vi "robotTurningAroundBall.vi"(7 "Game":refnum<class "Game.lvclass">, 8 "error in (no error)":errorcluster, 9 "Target":dbl[](array[numeric]), 10 "Robot in":refnum<class "Robot.lvclass">, 11 "KickToSkill in":refnum<class "KickToSkill.lvclass">) -> (0 "error out":errorcluster, 2 "Robot out":refnum<class "Robot.lvclass">, 3 "KickToSkill out":refnum<class "KickToSkill.lvclass">)   [LabVIEW 2021, in "KickToSkill.lvclass"]
uses:
  KickToSkill.lvclass
  Game_class/Game.lvclass
  Robot_class/Robot.lvclass
  robotTurningBallStates.ctl
  Object_class/Object.lvclass/Object.ctl
  Game_class/Game.lvclass/Game.ctl
  Robot_class/Robot.lvclass/Robot.ctl
  <vilib>/Analysis/baseanly.llb/Unit Vector (DBL).vi
  <vilib>/Analysis/coordinate.llb/2D Cartesian Coordinate Rotation (Scalar).vi
  Robot_class/Read orientation.vi
  Robot_class/Read dest_orientation.vi
  Robot_class/Read dest_x.vi
  Robot_class/Read dest_y.vi
  Game_class/Read BallRef.vi
  Object_class/Read position(x,y).vi
  Object_class/Read x.vi
  Robot_class/Write dest_orientation.vi
  Robot_class/Write dest_x.vi
  Robot_class/Write dest_y.vi
  Robot_class/Write kick_x.vi
  Robot_class/Write dribble.vi
  Ball_class/Ball.lvclass
  <vilib>/Analysis/NI_AALPro.lvlib
  <vilib>/Analysis/NI_AALBase.lvlib
panel:
  in  "Raio":dbl=123.0
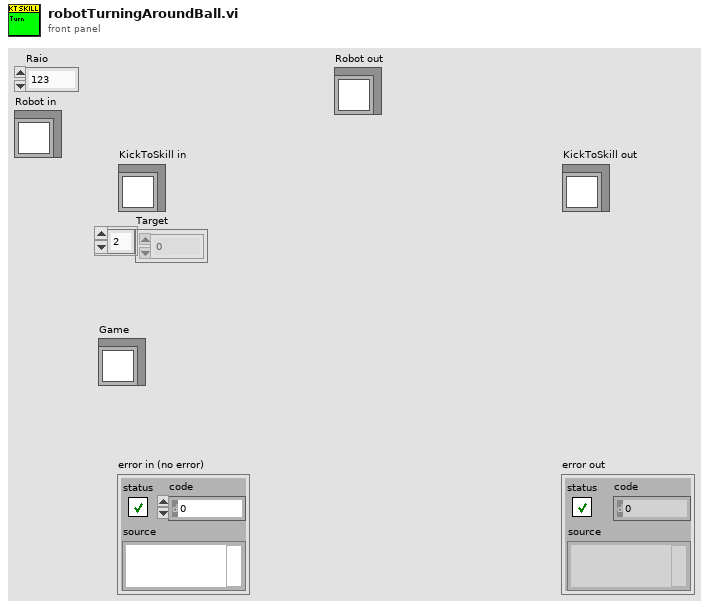
[diagram p1: front panel]
types:
  T1 = typedef "KickToSkill.lvclass/robotTurningBallStates.ctl" = enum16{"go straight to the target", "go to point A", "circulating the ball", "lining up", "shoot"}
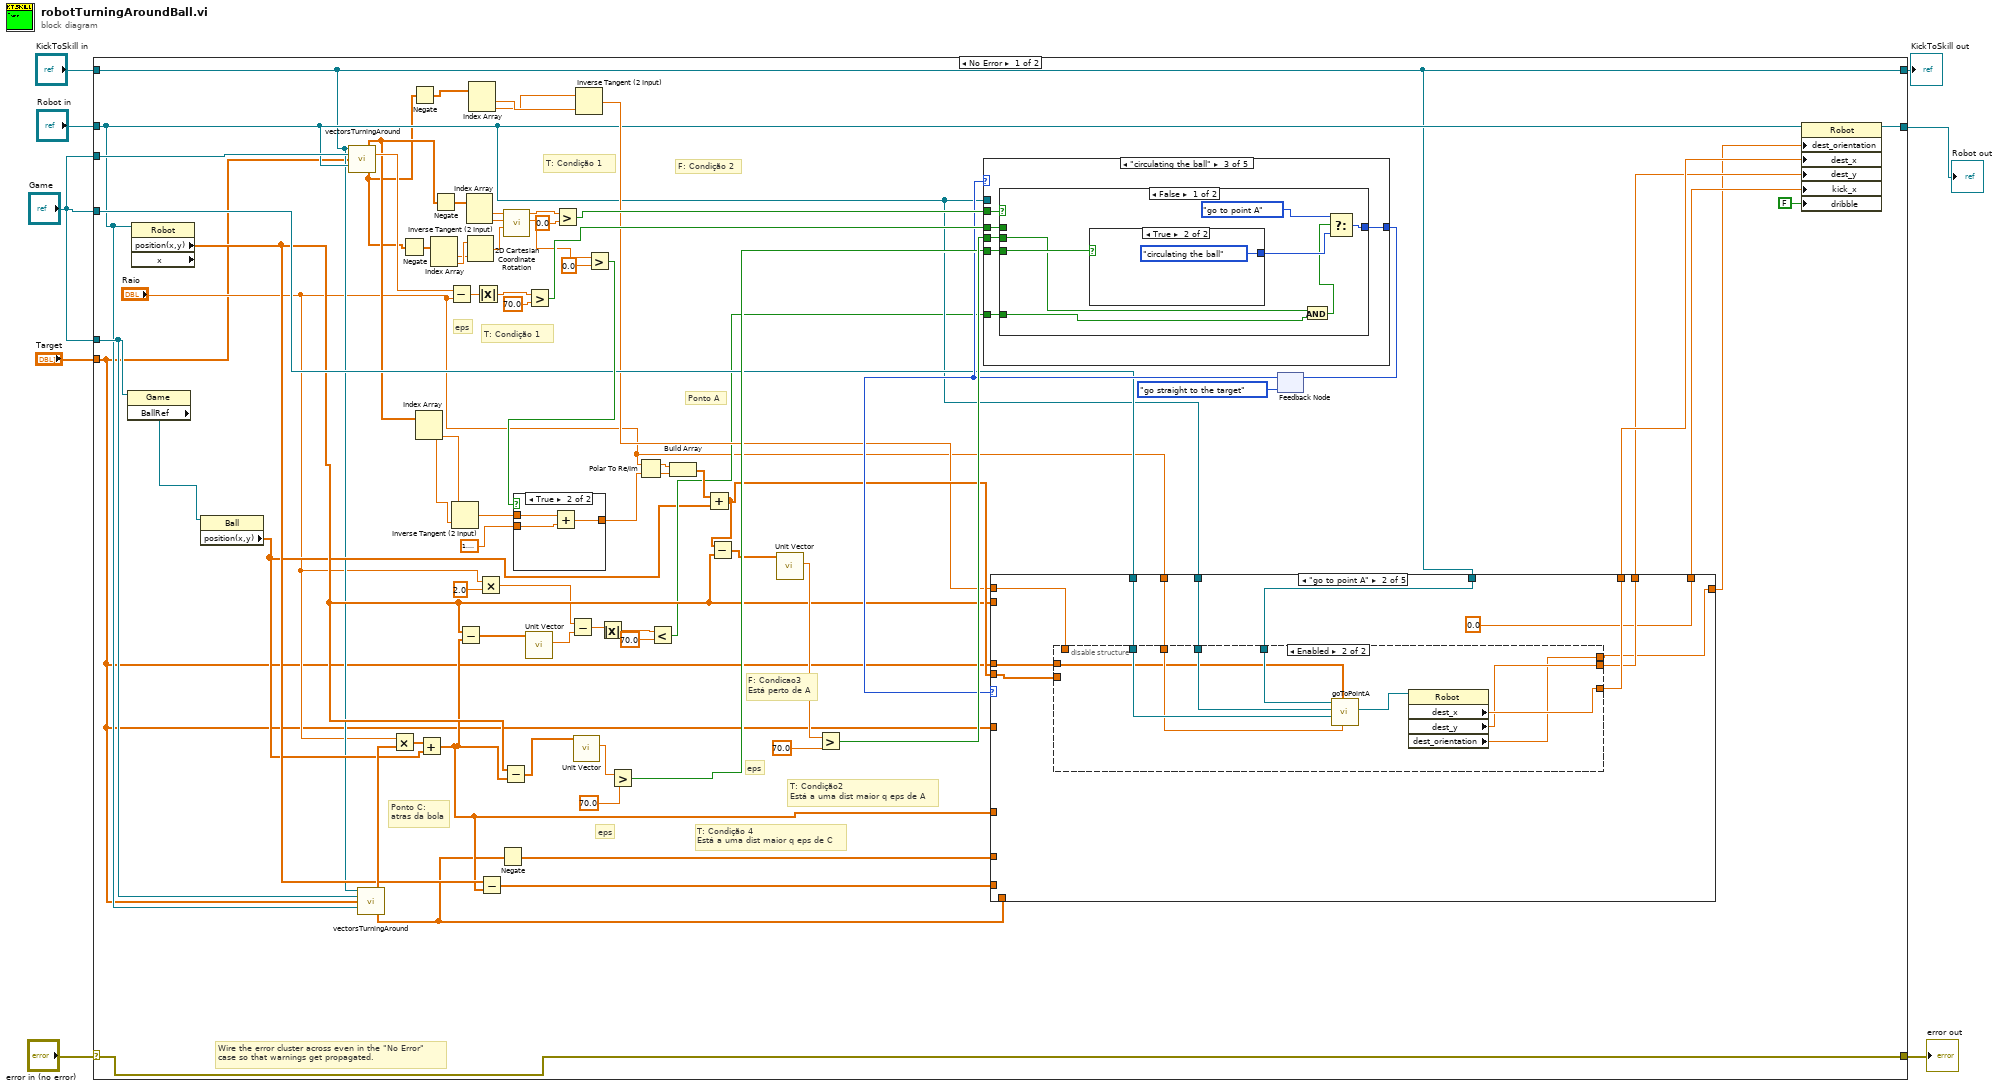
[diagram p0: block diagram]
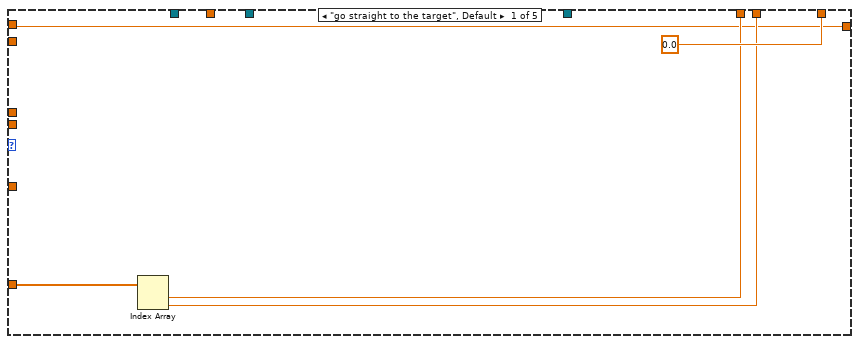
[diagram p2: hidden frame]
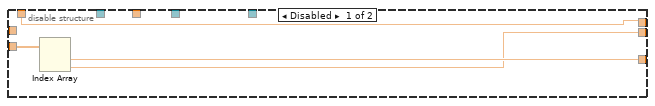
[diagram p3: hidden frame]
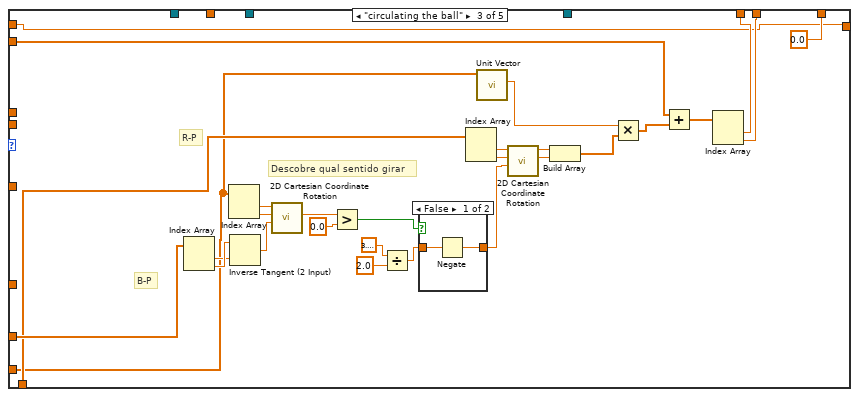
[diagram p4: hidden frame]
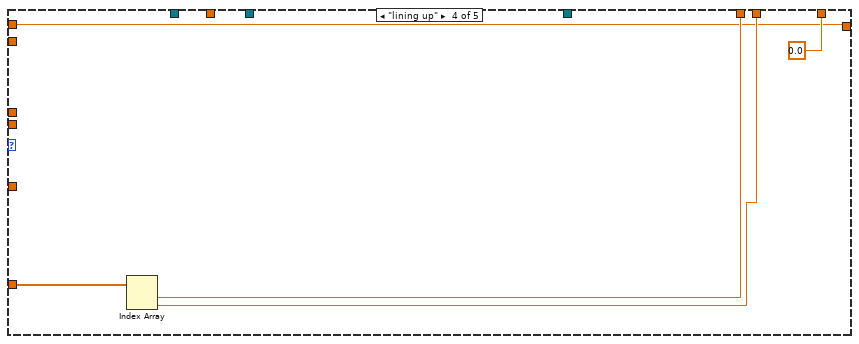
[diagram p6: hidden frame]
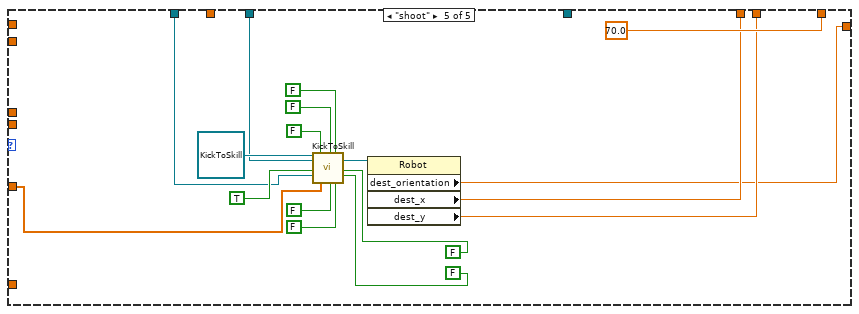
[diagram p7: hidden frame]
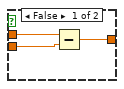
[diagram p8: hidden frame]
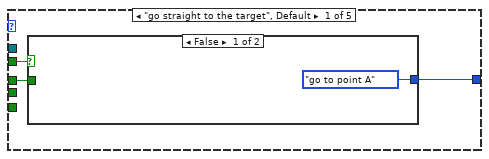
[diagram p9: hidden frame]
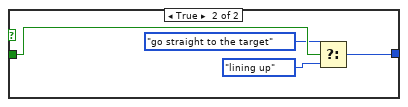
[diagram p10: hidden frame]
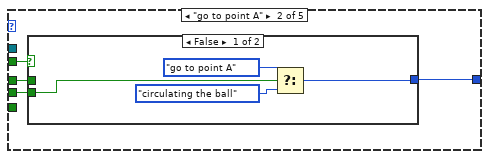
[diagram p11: hidden frame]
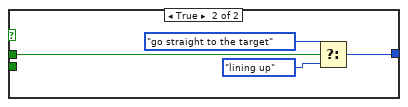
[diagram p12: hidden frame]
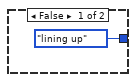
[diagram p13: hidden frame]
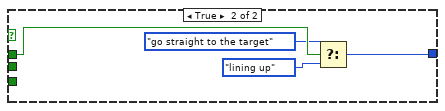
[diagram p14: hidden frame]
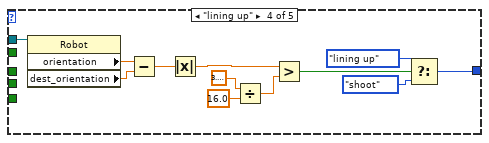
[diagram p15: hidden frame]
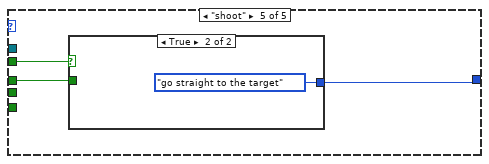
[diagram p16: hidden frame]
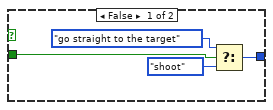
[diagram p17: hidden frame]
diagram:
  n1 = case shown="No Error" "error in (no error)" {
    selector: "error in (no error)" -> [w83 w233]
    tunnel: [w83 w233] -> w7
    tunnel: [w11 w232] -> w5
    tunnel: "KickToSkill in" -> [w11 w232]
    tunnel: "Robot in" -> [w29 w231]
    tunnel: [w82 w231] -> w3
    tunnel: "Target" -> [w9 _]
    tunnel: "Game" -> [w79 _]
    tunnel: "Game" -> [w30 _]
    tunnel: "Game" -> [w34 _]
    frame No Error {
      # "T: Condição 4\nEstá a uma dist maior q eps de C"
      # "F: Condicao3\nEstá perto de A"
      # "eps"
      # "Ponto C:\natras da bola"
      # "eps"
      # "eps"
      # "F: Condição 2"
      # "T: Condição2\nEstá a uma dist maior q eps de A"
      # "Ponto A"
      # "T: Condição 1"
      # "T: Condição 1"
      # "Wire the error cluster across even in the \"No Error\"\ncase so that warnings get propagated."
      n2 = property class="Game"(reference=w30) -> ("BallRef"=w53:refnum<class "Ball.lvclass">)  [unwired: 1 in, 2 out]
      n3 = property class="Robot" props=["position(x,y)", "x"](reference=w29) -> ("position(x,y)"=w27:dbl[])  [unwired: 1 in, 3 out]
      n4 = property class="Ball"(reference=w53) -> ("position(x,y)"=w14:dbl[])  [unwired: 1 in, 2 out]
      n5 = call "vectorsTurningAround.vi"("KickToSkill in"=w11, "Game"=w79, "Target"=w9, "Robot in"=w29) -> ("B-T"=w17:dbl[], "R-B norm"=w68:dbl, "R-B"=w16:dbl[])  [unwired: 4 in, 5 out]
      n6 = call "vectorsTurningAround.vi"("KickToSkill in"=w11, "Game"=w30, "Target"=w9, "Robot in"=w29) -> ("B-T"=w54:dbl[], "R-B"=w13:dbl[])  [unwired: 4 in, 6 out]
      n7 = Multiply(x="Raio", y=w54) -> (x*y=w52:dbl[])
      n8 = Negate(x=w16) -> (-x=w15:dbl[])
      n9 = Negate(x=w16) -> (-x=w28:dbl[])
      n10 = Index Array(array=w17) -> (element #1=w65:dbl, element #2=w64:dbl)  [unwired: 2 in]
      n11 = Add(x=w52, y=w14) -> (x+y=w26:dbl[])
      n12 = Index Array(array=w15) -> (element #1=w70:dbl, element #2=w71:dbl)  [unwired: 2 in]
      n13 = Negate(x=w17) -> (-x=w63:dbl[])
      n14 = Subtract(x=w68, y="Raio") -> (x-y=w76:dbl)
      n15 = Inverse Tangent (2 Input)(1:w65, 2:w64) -> (0:w62:dbl)
      n16 = Subtract(x=w27, y=w26) -> (x-y=w25:dbl[])
      n17 = Index Array(array=w63) -> (element #1=w72:dbl, element #2=w73:dbl)  [unwired: 2 in]
      n18 = Inverse Tangent (2 Input)(1:w70, 2:w71) -> (0:w69:dbl)
      n19 = Index Array(array=w28) -> (element #1=w41:dbl, element #2=w40:dbl)  [unwired: 2 in]
      n20 = Absolute Value(x=w76) -> (abs(x)=w77:dbl)
      n21 = Multiply(x="Raio", y=2.0) -> (x*y=w22:dbl)
      n22 = Subtract(x=w27, y=w26) -> (x-y=w35:dbl[])
      n23 = Negate(x=w13) -> (-x=w12:dbl[])
      n24 = Subtract(x=w27, y=w26) -> (x-y=w42:dbl[])
      n25 = call-poly <vilib>:"2D Cartesian Coordinate Rotation.vi"("theta"=w69, "y"=w73, "x"=w72) -> ("y out"=w60:dbl, "x out"=w74:dbl)  [unwired: 6 in, 1 out]
      n26 = call-poly <vilib>:"Unit Vector.vi"("Input Vector"=w25) -> ("norm"=w24:dbl)  [unwired: 8 in, 2 out]
      n27 = Greater?(x=w77, y=70.0) -> (0:w66:bool)
      n28 = Greater?(x=w74, y=0.0) -> (0:w67:bool)
      n29 = Subtract(x=w22, y=w24) -> (x-y=w21:dbl)
      n30 = call-poly <vilib>:"Unit Vector.vi"("Input Vector"=w42) -> ("norm"=w49:dbl)  [unwired: 8 in, 2 out]
      n31 = Inverse Tangent (2 Input)(1:w41, 2:w40) -> (0:w32:dbl)
      n32 = Greater?(x=w60, y=0.0) -> (0:w58:bool)
      n33 = case shown="True" w58 {
        tunnel: w62 -> [w167 w171]
        tunnel: 1.5707963267948966 -> [w168 w170]
        tunnel: [w166 w169] -> w47
        frame False {
          n34 = Subtract(x=w167, y=w168) -> (x-y=w166:dbl)
        }
        frame True {
          n35 = Add(x=w171, y=w170) -> (x+y=w169:dbl)
        }
      }
      n36 = Absolute Value(x=w21) -> (abs(x)=w20:dbl)
      n37 = Greater?(x=w49, y=70.0) -> (0:w50:bool)
      n38 = Polar To Re/Im(2:w47, 3:"Raio") -> (0:w45:dbl, 1:w46:dbl)
      n39 = Less?(x=w20, y=70.0) -> (x < y?=w18:bool)
      n40 = Build Array(w46, w45) -> (w44:dbl[])
      n41 = Add(x=w44, y=w14) -> (x+y=w43:dbl[])
      n42 = Subtract(x=w43, y=w27) -> (x-y=w31:dbl[])
      n43 = call-poly <vilib>:"Unit Vector.vi"("Input Vector"=w31) -> ("norm"=w56:dbl)  [unwired: 8 in, 2 out]
      n44 = Greater?(x=w56, y=70.0) -> (0:w55:bool)
      n45 = feedback #1(robotTurningBallStates."go straight to the target") -> (w48:T1)
      n46 = case shown="\"circulating the ball\"" w48 {
        tunnel: [w172 w181 w195 w211 w225] -> w81
        tunnel: w67 -> [w174 w183 w197 _ w224]
        tunnel: w66 -> [w173 w182 w196 _ w223]
        tunnel: w55 -> [_ w180 w194 _ _]
        tunnel: w50 -> [_ _ w193 _ _]
        tunnel: w29 -> [_ _ _ w222 _]
        tunnel: w18 -> [_ _ w192 _ _]
        frame "go straight to the target", Default {
          n47 = case shown="False" w174 {
            tunnel: w173 -> [_ w179]
            tunnel: [robotTurningBallStates."go to point A" w177] -> w172
            frame False {
            }
            frame True {
              n48 = Select(t=robotTurningBallStates."go straight to the target", s=w179, f=robotTurningBallStates."lining up") -> (s? t:f=w177:T1)
            }
          }
        }
        frame "go to point A" {
          n49 = case shown="False" w183 {
            tunnel: w182 -> [_ w191]
            tunnel: [w184 w189] -> w181
            tunnel: w180 -> [w187 _]
            frame False {
              n50 = Select(t=robotTurningBallStates."go to point A", s=w187, f=robotTurningBallStates."circulating the ball") -> (s? t:f=w184:T1)
            }
            frame True {
              n51 = Select(t=robotTurningBallStates."go straight to the target", s=w191, f=robotTurningBallStates."lining up") -> (s? t:f=w189:T1)
            }
          }
        }
        frame "circulating the ball" {
          n52 = case shown="False" w197 {
            tunnel: w196 -> [_ w210]
            tunnel: [w202 w208] -> w195
            tunnel: w194 -> [w200 _]
            tunnel: w193 -> [w201 _]
            tunnel: w192 -> [w199 _]
            frame False {
              n53 = case shown="True" w201 {
                tunnel: [robotTurningBallStates."lining up" robotTurningBallStates."circulating the ball"] -> w203
                frame False {
                }
                frame True {
                }
              }
              n54 = And(x=w200, y=w199) -> (x .and. y?=w198:bool)
              n55 = Select(t=robotTurningBallStates."go to point A", s=w198, f=w203) -> (s? t:f=w202:T1)
            }
            frame True {
              n56 = Select(t=robotTurningBallStates."go straight to the target", s=w210, f=robotTurningBallStates."lining up") -> (s? t:f=w208:T1)
            }
          }
        }
        frame "lining up" {
          n57 = property class="Robot"(reference=w222) -> ("orientation"=w221:dbl, "dest_orientation"=w220:dbl)  [unwired: 1 in, 2 out]
          n58 = Subtract(x=w221, y=w220) -> (x-y=w219:dbl)
          n59 = Absolute Value(x=w219) -> (abs(x)=w218:dbl)
          n60 = Divide(x=3.141592653589793, y=16.0) -> (x/y=w215:dbl)
          n61 = Greater?(x=w218, y=w215) -> (0:w214:bool)
          n62 = Select(t=robotTurningBallStates."lining up", s=w214, f=robotTurningBallStates."shoot") -> (s? t:f=w211:T1)
        }
        frame "shoot" {
          n63 = case shown="True" w224 {
            tunnel: w223 -> [w229 _]
            tunnel: [w227 robotTurningBallStates."go straight to the target"] -> w225
            frame False {
              n64 = Select(t=robotTurningBallStates."go straight to the target", s=w229, f=robotTurningBallStates."shoot") -> (s? t:f=w227:T1)
            }
            frame True {
            }
          }
        }
      }
      n65 = case shown="\"go to point A\"" w48 {
        tunnel: w43 -> [_ w99 _ _ _]
        tunnel: [0.0 ("kick_x") 0.0 ("kick_x") 0.0 ("kick_x") 0.0 ("kick_x") 70.0 ("kick_x")] -> w38
        tunnel: w26 -> [w87 _ _ w147 _]
        tunnel: [w86 w98 w115 w146 w151] -> w37
        tunnel: [w85 w97 w114 w145 w150] -> w36
        tunnel: w12 -> [_ _ w123 _ _]
        tunnel: w35 -> [_ _ w121 _ _]
        tunnel: w13 -> [_ _ w122 _ _]
        tunnel: w27 -> [_ _ w118 _ _]
        tunnel: w9 -> [_ _ _ _ w155]
        tunnel: w29 -> [_ w95 _ _ w154]
        tunnel: w34 -> [_ w94 _ _ w153]
        tunnel: w32 -> [w84 w89 w113 w144 _]
        tunnel: [w84 w90 w113 w144 w149] -> w33
        tunnel: w11 -> [_ w96 _ _ _]
        tunnel: "Raio" -> [_ w93 _ _ _]
        tunnel: w9 -> [_ w92 _ _ _]
        frame "go straight to the target", Default {
          n66 = Index Array(array=w87) -> (element #1=w86:dbl, element #2=w85:dbl)  [unwired: 2 in]
        }
        frame "go to point A" {
          n67 = disable-structure shown="Enabled" {
            disable-tunnel: w99 -> [w103 _]
            disable-tunnel: [w102 w106] -> w98
            disable-tunnel: [w101 w105] -> w97
            disable-tunnel: w96 -> [_ w112]
            disable-tunnel: w95 -> [_ w111]
            disable-tunnel: w94 -> [_ w110]
            disable-tunnel: w93 -> [_ w109]
            disable-tunnel: w92 -> [_ w108]
            disable-tunnel: [w100 w104] -> w90
            disable-tunnel: w89 -> [w100 _]
            frame Disabled {
              n68 = Index Array(array=w103) -> (element #1=w102:dbl, element #2=w101:dbl)  [unwired: 2 in]
            }
            frame Enabled {
              n69 = call "goToPointA.vi"("Raio"=w109, "Target"=w108, "Game"=w110, "Robot in"=w111, "KickToSkill in"=w112) -> ("Robot out"=w107:refnum<class "Robot.lvclass">)  [unwired: 4 in, 2 out]
              n70 = property class="Robot"(reference=w107) -> ("dest_x"=w106:dbl, "dest_y"=w105:dbl, "dest_orientation"=w104:dbl)  [unwired: 1 in, 2 out]
            }
          }
        }
        frame "circulating the ball" {
          # "B-P"
          # "R-P"
          # "Descobre qual sentido girar"
          n71 = Index Array(array=w123) -> (element #1=w124:dbl, element #2=w125:dbl)  [unwired: 2 in]
          n72 = Index Array(array=w121) -> (element #1=w131:dbl, element #2=w130:dbl)  [unwired: 2 in]
          n73 = Inverse Tangent (2 Input)(1:w124, 2:w125) -> (0:w129:dbl)
          n74 = call-poly <vilib>:"2D Cartesian Coordinate Rotation.vi"("theta"=w129, "y"=w130, "x"=w131) -> ("y out"=w128:dbl)  [unwired: 6 in, 2 out]
          n75 = Greater?(x=w128, y=0.0) -> (0:w126:bool)
          n76 = Divide(x=3.141592653589793, y=2.0) -> (x/y=w133:dbl)
          n77 = case shown="False" w126 {
            tunnel: w133 -> [w142 w143]
            tunnel: [w141 w143] -> w132
            frame False {
              n78 = Negate(x=w142) -> (-x=w141:dbl)
            }
            frame True {
            }
          }
          n79 = Index Array(array=w122) -> (element #1=w139:dbl, element #2=w138:dbl)  [unwired: 2 in]
          n80 = call-poly <vilib>:"Unit Vector.vi"("Input Vector"=w121) -> ("norm"=w120:dbl)  [unwired: 8 in, 2 out]
          n81 = call-poly <vilib>:"2D Cartesian Coordinate Rotation.vi"("theta"=w132, "y"=w138, "x"=w139) -> ("y out"=w136:dbl, "x out"=w137:dbl)  [unwired: 6 in, 1 out]
          n82 = Build Array(w137, w136) -> (w119:dbl[])
          n83 = Multiply(x=w120, y=w119) -> (x*y=w117:dbl[])
          n84 = Add(x=w118, y=w117) -> (x+y=w116:dbl[])
          n85 = Index Array(array=w116) -> (element #1=w115:dbl, element #2=w114:dbl)  [unwired: 2 in]
        }
        frame "lining up" {
          n86 = Index Array(array=w147) -> (element #1=w146:dbl, element #2=w145:dbl)  [unwired: 2 in]
        }
        frame "shoot" {
          n87 = call "KickToSkill.vi"("KickToSkill in"=refnum<class "KickToSkill.lvclass"> refnum, "Robot"=w154, "firstCall?"=TRUE, "Game"=w153, "use criteria?"=FALSE, "Target"=w155, "chipKick ?"=FALSE, "KickForce 0?"=FALSE, "WeakKick"=FALSE, "ForceInGame"=FALSE, "IgnorePosEst"=FALSE, "pass?"=FALSE) -> ("Robot out"=w157:refnum<class "Robot.lvclass">)  [unwired: 4 in, 3 out]
          n88 = property class="Robot"(reference=w157) -> ("dest_orientation"=w149:dbl, "dest_x"=w151:dbl, "dest_y"=w150:dbl)  [unwired: 1 in, 2 out]
        }
      }
      n89 = feedback-in #1(w81) -> ()
      n90 = property class="Robot"(reference=w29, "dest_orientation"=w33, "dest_x"=w37, "dest_y"=w36, "kick_x"=w38, "dribble"=FALSE) -> (reference out=w82:refnum<class "Robot.lvclass">)  [unwired: 1 in, 1 out]
    }
    frame Error {
    }
  }
  "error out" <- w7
  "KickToSkill out" <- w5
  "Robot out" <- w3
